vi "_openIE.vi"(8 "error in (no error)":errorcluster, 11 "URL":string="www.ni.com/dataplugins") -> (0 "error out":errorcluster, 3 "URL out":string)   [LabVIEW 2017]
doc: "This VI uses ActiveX to open IE in its own window and point it to the URL typed into the string control."
panel:
  in  "SHDocVw.IWebBrowser2":refnum<k7>
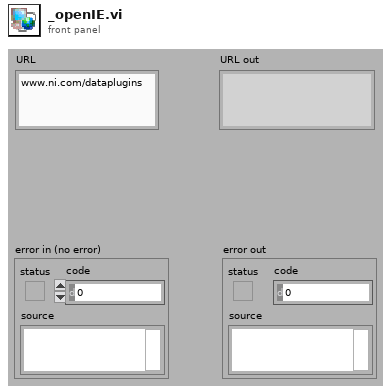
[diagram p1: front panel]
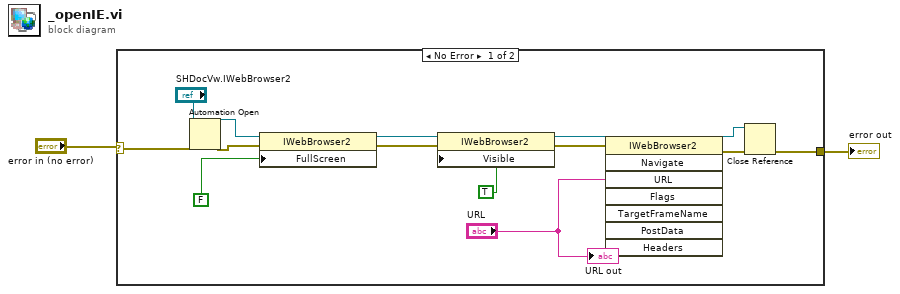
[diagram p0: block diagram]
diagram:
  n1 = case shown="No Error" "error in (no error)" {
    selector: "error in (no error)" -> [w3 w17]
    tunnel: [w4 w17] -> w2
    frame No Error {
      n2 = Automation Open(error in (no error)=w3, Automation Refnum="SHDocVw.IWebBrowser2") -> (Automation Refnum=w16:refnum<k7>, error out=w15:errorcluster)  [unwired: 2 out]
      n3 = property class="IWebBrowser2"(reference=w16, error in=w15, "FullScreen"=FALSE) -> (reference out=w7:refnum<k7>, error out=w6:errorcluster)
      n4 = property class="IWebBrowser2"(reference=w7, error in=w6, "Visible"=TRUE) -> (reference out=w12:refnum<k7>, error out=w13:errorcluster)
      n5 = invoke class="IWebBrowser2" method="Navigate"(reference=w12, error in=w13, "URL"="URL") -> (reference out=w9:refnum<k7>, error out=w10:errorcluster)  [unwired: 5 in, 6 out]
      n6 = Close Reference(reference=w9, error in (no error)=w10) -> (error out=w4:errorcluster)
      "URL out" <- "URL"
    }
    frame Error {
    }
  }
  "error out" <- w2
